vi "HEWH Display Message.vi"(6 "Station ID":T1, 7 "Display Message Location":T2, 8 "Error In":errorcluster, 9 "Terminate Condition Input":string, 10 "Purge Time (Seconds)":dbl, 11 "Purge Elapsed Time":dbl format="%.2f") -> (0 "Error Out":errorcluster, 2 "Message":string)   [LabVIEW 2016]
uses:
  Type Definitions/User Message.ctl
  Custom Instrument Control/MW100/Type Definitions/Station ID Selector.ctl
  Utility/Custom Pallet Controls/Custom Pallet String.ctl
panel:
  # "Purge Condtion"
  # "Terminate Conditions"
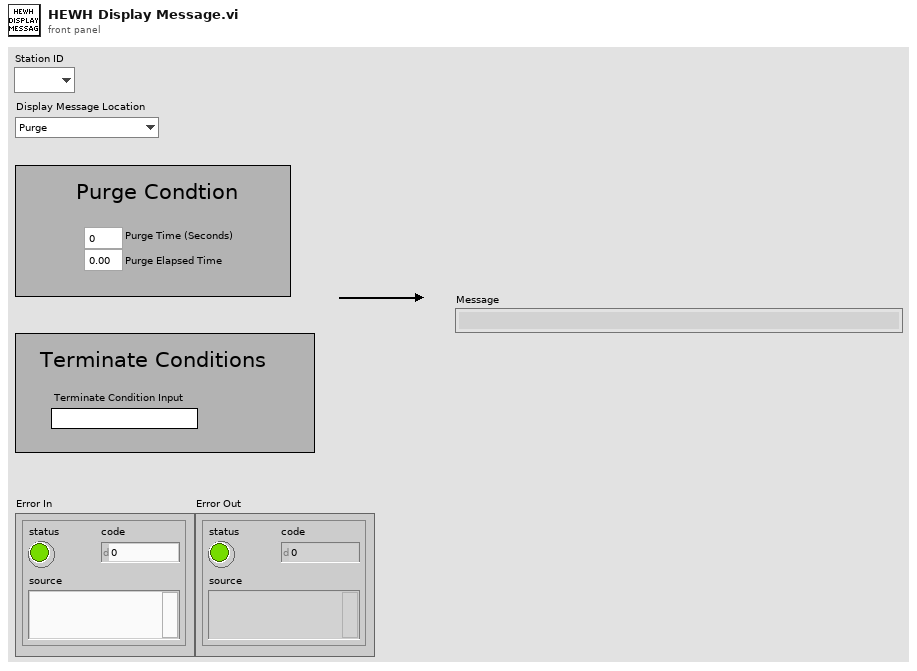
[diagram p1: front panel]
types:
  T1 = typedef "Station ID Selector.ctl" = enum16{"", "A", "B", "C", "D", "Global"}
  T2 = typedef "User Message.ctl" = enum16{"Purge", "Drawing", "PRAT"}
  T3 = typedef "Custom Pallet String.ctl" = string
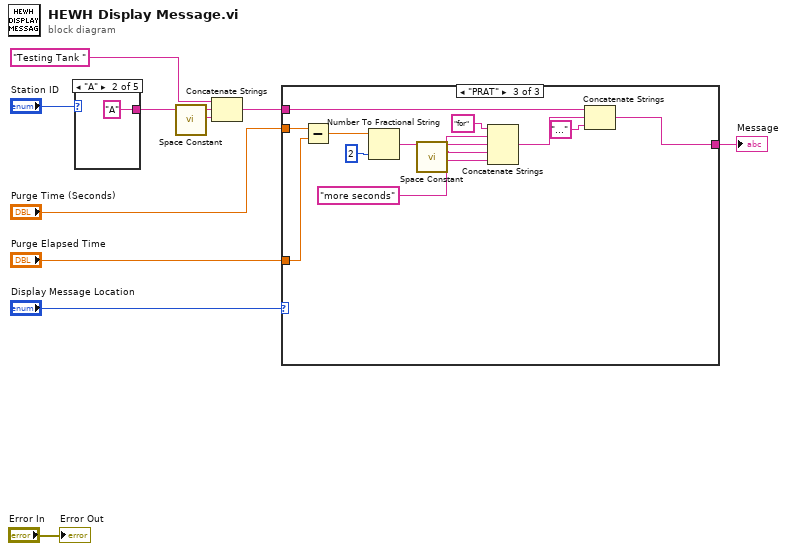
[diagram p0: block diagram]
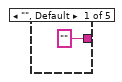
[diagram p2: hidden frame]
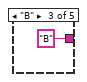
[diagram p3: hidden frame]
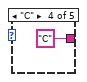
[diagram p4: hidden frame]
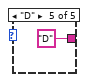
[diagram p5: hidden frame]
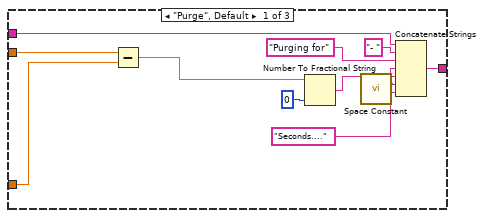
[diagram p6: hidden frame]
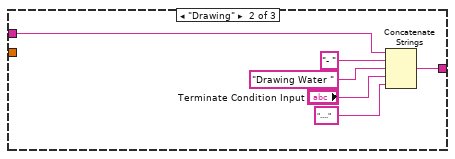
[diagram p7: hidden frame]
diagram:
  n1 = case shown="\"A\"" "Station ID" {
    tunnel: ["" "A" "B" "C" "D"] -> w6
    frame "", Default {
    }
    frame "A" {
    }
    frame "B" {
    }
    frame "C" {
    }
    frame "D" {
    }
  }
  n2 = call <vilib>:"Space Constant.vi"() -> ("String"=w5:string)
  n3 = Concatenate Strings("Testing Tank " ("string"), w6, w5) -> (w2:string)
  n4 = case shown="\"PRAT\"" "Display Message Location" {
    tunnel: [w26 w29 w34] -> w10
    tunnel: "Purge Time (Seconds)" -> [w19 _ w38]
    tunnel: "Purge Elapsed Time" -> [w18 _ w37]
    tunnel: w2 -> [w17 w28 w33]
    frame "Purge", Default {
      n5 = Subtract(x=w19, y=w18) -> (x-y=w20:dbl)
      n6 = Number To Fractional String(number=w20, precision (6)=i16 0) -> (F-format string=w22:string)  [unwired: 2 in]
      n7 = call <vilib>:"Space Constant.vi"() -> ("String"=w24:string)
      n8 = Concatenate Strings(w17, "- " ("string"), T3 "Purging for" ("Message"), w24, w22, w24, "Seconds...." ("string")) -> (w26:string)
    }
    frame "Drawing" {
      n9 = Concatenate Strings(w28, "- " ("string"), T3 "Drawing Water " ("Message"), "Terminate Condition Input", "...." ("string")) -> (w29:string)
    }
    frame "PRAT" {
      n10 = Subtract(x=w38, y=w37) -> (x-y=w39:dbl)
      n11 = Number To Fractional String(number=w39, precision (6)=i16 2) -> (F-format string=w42:string)  [unwired: 2 in]
      n12 = call <vilib>:"Space Constant.vi"() -> ("String"=w43:string)
      n13 = Concatenate Strings("for", w43, w42, w43, "more seconds" ("string")) -> (w35:string)
      n14 = Concatenate Strings(w33, w35, "...") -> (w34:string)
    }
  }
  "Message" <- w10
  "Error Out" <- "Error In"
